vi "EncodeUInt16.vi"(1 "Data In":u16[](array[numeric])) -> (0 "Data Out":u8[](array[numeric]))   [LabVIEW 2014, in "navX-MXP IMU.lvlib"]
uses:
  navX-MXP IMU.lvlib
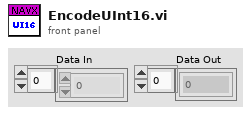
[diagram p1: front panel]
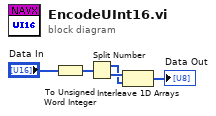
[diagram p0: block diagram]
diagram:
  n1 = To Unsigned Word Integer(number="Data In") -> (unsigned 16bit integer=w1:u16[])
  n2 = Split Number(x=w1) -> (hi(x)=w4:u8[], lo(x)=w5:u8[])
  n3 = Interleave 1D Arrays(w5, w4) -> (→"Data Out":u8[])
